vi "Is Empty Object.vi"(1 "Value in":variant) -> (0 "Is Empty Object?":bool)   [LabVIEW 2019, in "JSON.lvlib"]
doc: "Returns <b>True</b> if the <b>Value in</b> is a Cluster with the U16 Enum <b>\"empty\"</b> placeholder.\n\nCreated by: Ryan Pacini"
uses:
  JSON.lvlib
  <vilib>/Utility/Data Type/NI_Data Type.lvlib
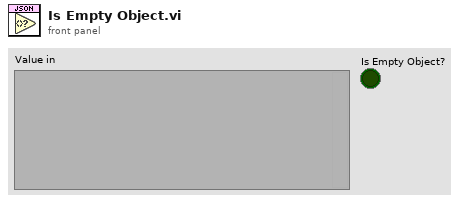
[diagram p1: front panel]
types:
  T1 = typedef "NI_Data Type.lvlib/Data Type.ctl" = enum8{"Invalid Type", "Void", "I8", "I16", "I32", "I64", "U8", "U16", "U32", "U64", "Single Float", "Double Float", "Extended Float", "Single Complex", "Double Complex", "Extended Complex", "Enum U8", "Enum U16", "Enum U32", "Enum U64", "Single Float With Unit", "Double Float With Unit", "Extended Float With Unit", "Single Complex with Unit", "Double Complex with Unit", "Extended Complex with Unit", "Boolean", "String", "Path", "Picture", "Tag", "Array", "Cluster", "Variant", "LV Variant", "Waveform", "Timestamp", "Digital Waveform", "Digital Data", "ExpressData", "Refnum", "External Data", "VI", "Poly VI", "LabVIEW Class Instance", "Fixed Point", "Set Collection", "Map Collection"}
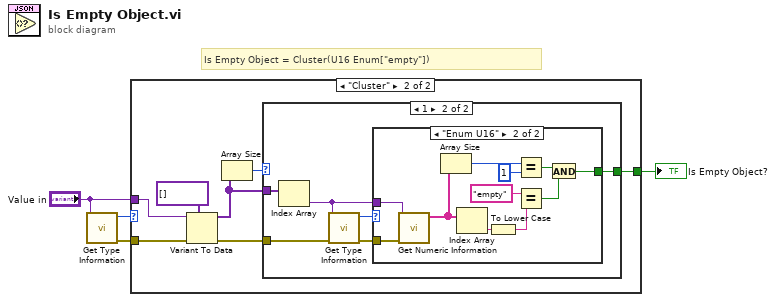
[diagram p0: block diagram]
diagram:
  # "Is Empty Object = Cluster(U16 Enum[\"empty\"])"
  n1 = call <vilib>:"Get Type Information.vi"("variant"="Value in") -> ("error out"=w4:errorcluster, "type"=w3:T1)  [unwired: 6 in, 3 out]
  n2 = case shown="\"Cluster\"" w3 {
    tunnel: w4 -> [_ w11]
    tunnel: "Value in" -> [_ w10]
    tunnel: [_ w5] -> w1
    frame Default {
    }
    frame "Cluster" {
      n3 = Variant To Data(error in=w11, type=variant[] [], Variant=w10) -> (data=w6:variant[], error out=w8:errorcluster)
      n4 = Array Size(array=w6) -> (size(s)=w7:i32)
      n5 = case shown="1" w7 {
        tunnel: w8 -> [_ w17]
        tunnel: w6 -> [_ w16]
        tunnel: [_ w12] -> w5
        frame 0, Default {
        }
        frame 1 {
          n6 = Index Array(array=w16) -> (element=w13:variant)  [unwired: 1 in]
          n7 = call <vilib>:"Get Type Information.vi"("error in (no error)"=w17, "variant"=w13) -> ("error out"=w14:errorcluster, "type"=w15:T1)  [unwired: 5 in, 3 out]
          n8 = case shown="\"Enum U16\"" w15 {
            tunnel: w14 -> [_ w28]
            tunnel: w13 -> [_ w27]
            tunnel: [_ w18] -> w12
            frame "Invalid Type", Default {
            }
            frame "Enum U16" {
              n9 = call <vilib>:"Get Numeric Information.vi"("error in (no error)"=w28, "variant"=w27) -> ("enum names"=w24:string[])  [unwired: 6 in, 3 out]
              n10 = Array Size(array=w24) -> (size(s)=w26:i32)
              n11 = Index Array(array=w24) -> (element=w23:string)  [unwired: 1 in]
              n12 = To Lower Case(string=w23) -> (all lower case string=w21:string)
              n13 = Equal?(x=w26, y=1) -> (x = y?=w19:bool)
              n14 = Equal?(x="empty" ("y"), y=w21) -> (x = y?=w20:bool)
              n15 = And(x=w19, y=w20) -> (x .and. y?=w18:bool)
            }
          }
        }
      }
    }
  }
  "Is Empty Object?" <- w1
